vi "Overtilt warning.vi"(1 "Error In":errorcluster, 2 "Y":i16, 3 "X":i16) -> (0 "Error Out":errorcluster)   [LabVIEW 2015]
uses:
  Error.ctl
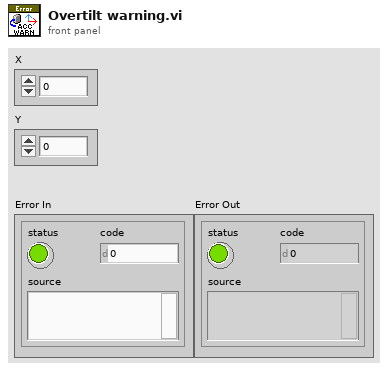
[diagram p1: front panel]
types:
  T1 = typedef "Error.ctl" = enum16{"No Error", "Custom", "Standard", "GPS Signal", "YH Left", "YL Right", "XL Back", "XH Front"}
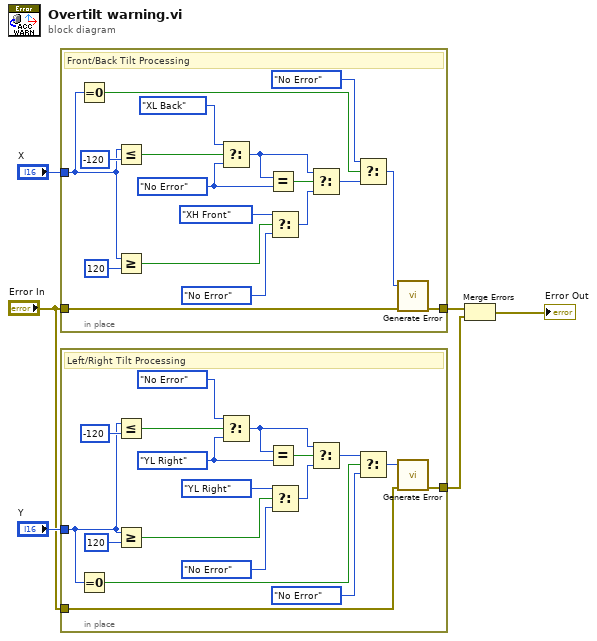
[diagram p0: block diagram]
diagram:
  n1 = in-place {
    in-place-border: [w24] -> w6
    in-place-border: "X" -> [w9]
    in-place-border: "Error In" -> [w7]
    w18 = Error."No Error" ("Enum")
    # "Front/Back Tilt Processing"
    n2 = Equal To 0?(x=w9) -> (x = 0?=w23:bool)
    n3 = Less Or Equal?(x=w9, y=i16 -120) -> (x <= y?=w13:bool)
    n4 = Greater Or Equal?(x=w9, y=i16 120) -> (x >= y?=w14:bool)
    n5 = Select(t=Error."XL Back" ("Enum"), s=w13, f=w18) -> (s? t:f=w20:T1)
    n6 = Equal?(x=w20, y=w18) -> (x = y?=w19:bool)
    n7 = Select(t=Error."XH Front" ("Enum"), s=w14, f=Error."No Error" ("Enum")) -> (s? t:f=w21:T1)
    n8 = Select(t=w20, s=w19, f=w21) -> (s? t:f=w22:T1)
    n9 = Select(t=Error."No Error", s=w23, f=w22) -> (s? t:f=w8:T1)
    n10 = call "Generate Error.vi"("Error In"=w7, "Enum"=w8) -> ("Error Out"=w24:errorcluster)  [unwired: 9 in]
  }
  n11 = in-place {
    in-place-border: "Y" -> [w30]
    in-place-border: [w29] -> w2
    in-place-border: "Error In" -> [w27]
    w39 = Error."YL Right" ("Enum")
    # "Left/Right Tilt Processing"
    n12 = Equal To 0?(x=w30) -> (x = 0?=w42:bool)
    n13 = Less Or Equal?(x=w30, y=i16 -120) -> (x <= y?=w33:bool)
    n14 = Greater Or Equal?(x=w30, y=i16 120) -> (x >= y?=w34:bool)
    n15 = Select(t=Error."No Error" ("Enum"), s=w33, f=w39) -> (s? t:f=w40:T1)
    n16 = Equal?(x=w40, y=w39) -> (x = y?=w38:bool)
    n17 = Select(t=Error."YL Right" ("Enum"), s=w34, f=Error."No Error" ("Enum")) -> (s? t:f=w41:T1)
    n18 = Select(t=w40, s=w38, f=w41) -> (s? t:f=w25:T1)
    n19 = Select(t=w25, s=w42, f=Error."No Error" ("t")) -> (s? t:f=w28:T1)
    n20 = call "Generate Error.vi"("Error In"=w27, "Enum"=w28) -> ("Error Out"=w29:errorcluster)  [unwired: 9 in]
  }
  n21 = Merge Errors "Merge Errors"(w6, w2) -> (→"Error Out":errorcluster)
